vi "Loader.vi"(1 "Down (Forward)":bool, 2 "Enum":enum16{"Start", "Run", "End"}(ring)) -> (0 "State":T1)   [LabVIEW 2014]
uses:
  TypeDefs/Solenoid Module 1.ctl
  <vilib>/Rock Robotics/WPI/Solenoid/WPI_SolenoidChannel.ctl
  <vilib>/Rock Robotics/SystemInterfaces/Typedef/FPGA_TypedefSolenoidModule.ctl
  <vilib>/Rock Robotics/WPI/Solenoid/WPI_SolenoidValue.ctl
  <vilib>/Rock Robotics/WPI/Solenoid/WPI_SolenoidOpenDouble.vi
  Team Code/Robot Global Data.vi
  <vilib>/Rock Robotics/WPI/Solenoid/WPI_SolenoidSetEnum.vi
panel:
  in  "Solenoid Module 1":T2={"Loader FWD"=enum."Solenoid 1", "Loader REV"=enum."Solenoid 2", "Climber"=enum."Solenoid 3", "Unassigned"=enum."Solenoid 4", "Unassigned"=enum."Solenoid 5", "Unassigned"=enum."Solenoid 6", "Unassigned"=enum."Solenoid 7", "Unassigned"=enum."Solenoid 7", "Module"=enum."Solenoid Module 1"}
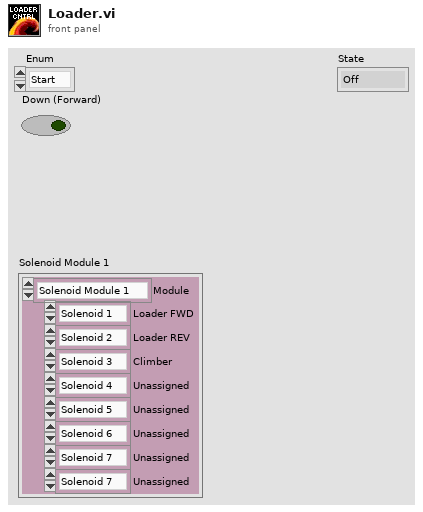
[diagram p1: front panel]
types:
  T1 = typedef "WPI_SolenoidValue.ctl" = enum16{"Off", "On", "Forward", "Reverse"}
  T2 = typedef "Solenoid Module 1.ctl" = cluster{"Loader FWD":T3, "Loader REV":T3, "Climber":T3, "Unassigned":T3, "Unassigned":T3, "Unassigned":T3, "Unassigned":T3, "Unassigned":T3, "Module":T4}
  T3 = typedef "WPI_SolenoidChannel.ctl" = enum8{"Solenoid 1", "Solenoid 2", "Solenoid 3", "Solenoid 4", "Solenoid 5", "Solenoid 6", "Solenoid 7", "Solenoid 8", "Invalid"}
  T4 = typedef "FPGA_TypedefSolenoidModule.ctl" = enum16{"Solenoid Module 1", "Solenoid Module 2"}
  T5 = enum16{"Nothing", "Load", "Lock", "Pass", "Grab", "Loader Down", "Shoot", "Auto Start", "Tele Start"}
  T6 = typedef "WPI_SolenoidDevRef.ctl" = cluster{"DevStatus":errorcluster, "Solenoid Module":T4, "Forward Solenoid Channel":T3, "Reverse Solenoid Channel":T3}
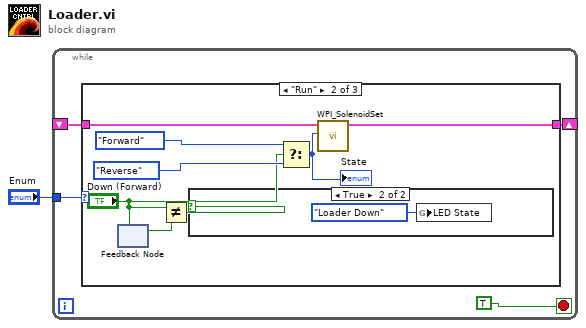
[diagram p0: block diagram]
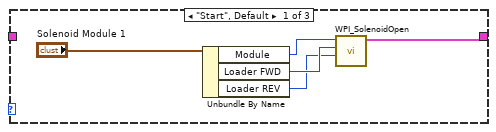
[diagram p2: hidden frame]
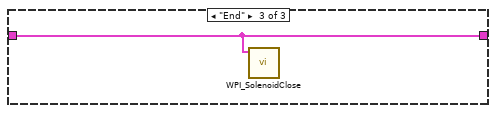
[diagram p4: hidden frame]
diagram:
  n1 = while {
    tunnel: "Enum" -> [w4]
    shift-right: [w2] -> _
    shift-left: _ -> [w3]
    stop <- TRUE stop-if-true
    n2 = case shown="\"Run\"" w4 {
      tunnel: w3 -> [_ w18 w20]
      tunnel: [w6 w17 w20] -> w2
      frame "Start", Default {
        n3 = Unbundle By Name("Solenoid Module 1") -> ("Module"=w9:T4, "Loader FWD"=w8:T3, "Loader REV"=w7:T3)
        n4 = call-poly <vilib>:"WPI_SolenoidOpen.vi"("Reverse Solenoid Channel"=w7, "Forward Solenoid Channel"=w8, "Solenoid Module (Module 1)"=w9) -> ("SolenoidDevRef"=w6:T6)  [unwired: 7 in, 1 out]
      }
      frame "Run" {
        n5 = feedback-in #1("Down (Forward)") -> ()
        n6 = feedback #1() -> (w13:bool)  [unwired: 1 in]
        n7 = Not Equal?(x="Down (Forward)", y=w13) -> (x != y?=w11:bool)
        n8 = case shown="True" w11 {
          frame False {
          }
          frame True {
            n9 = global write "Robot Global Data.vi" "LED State"(T5."Loader Down" ("LED State")) -> ()
          }
        }
        n10 = Select(t=WPI_SolenoidValue."Forward" ("Value"), s="Down (Forward)", f=WPI_SolenoidValue."Reverse" ("Value")) -> (s? t:f=w14:T1)
        "State" <- w14
        n11 = call-poly <vilib>:"WPI_SolenoidSet.vi"("Value"=w14, "SolenoidDevRef"=w18) -> ("SolenoidDevRef"=w17:T6)  [unwired: 8 in, 1 out]
      }
      frame "End" {
        n12 = call <vilib>:"WPI_SolenoidClose.vi"("SolenoidDevRef"=w20) -> ()  [unwired: 10 in, 1 out]
      }
    }
  }
